vi "Min Read Single.vi"(8 "error in":errorcluster, 9 "Channel Index":i32=1, 11 "Min Voltage Limit in":refnum<class "Voltage Limit.lvclass">) -> (0 "error out":errorcluster, 1 "Changed or First Call?":bool, 2 "Current Setpoint":dbl, 3 "Min Voltage Limit out":refnum<class "Voltage Limit.lvclass">)   [LabVIEW 2023, in "Voltage Limit.lvclass"]
uses:
  Voltage Limit.lvclass
  Parents/Limit/Limit.lvclass
  Voltage Limit.lvclass/Voltage Limit.ctl
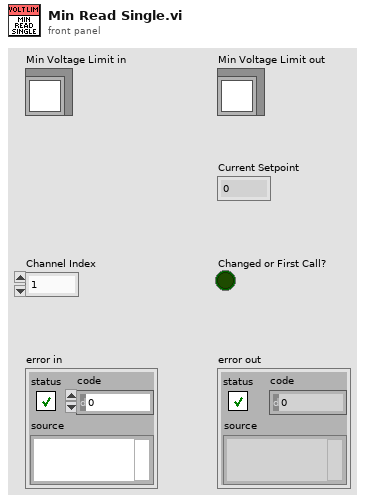
[diagram p1: front panel]
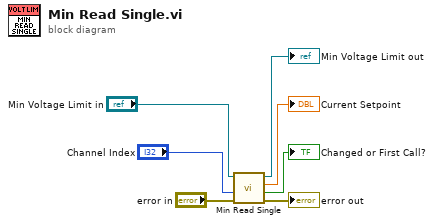
[diagram p0: block diagram]
diagram:
  n1 = call-parent "Min Read Single.vi"("error in"="error in", "Channel Index"="Channel Index", "Min Limit in"="Min Voltage Limit in") -> ("error out"=→"error out":errorcluster, "Changed or First Call?"=→"Changed or First Call?":bool, "Current Setpoint"=→"Current Setpoint":dbl, "Min Limit out"=→"Min Voltage Limit out":refnum<class "Voltage Limit.lvclass">)  [unwired: 5 in]
